vi "Operator error message space bar or print label.vi"(8 "error in (no error)":errorcluster, 11 "Message":string) -> (0 "error out":errorcluster, 3 "F1 Key hit?":bool)   [LabVIEW 2013]
uses:
  <vilib>/event_ctls.llb/eventvkey.ctl
panel:
  # "Operator Message"
  # "Press SPACE BAR to continue with no error label, else F1 key to print error label"
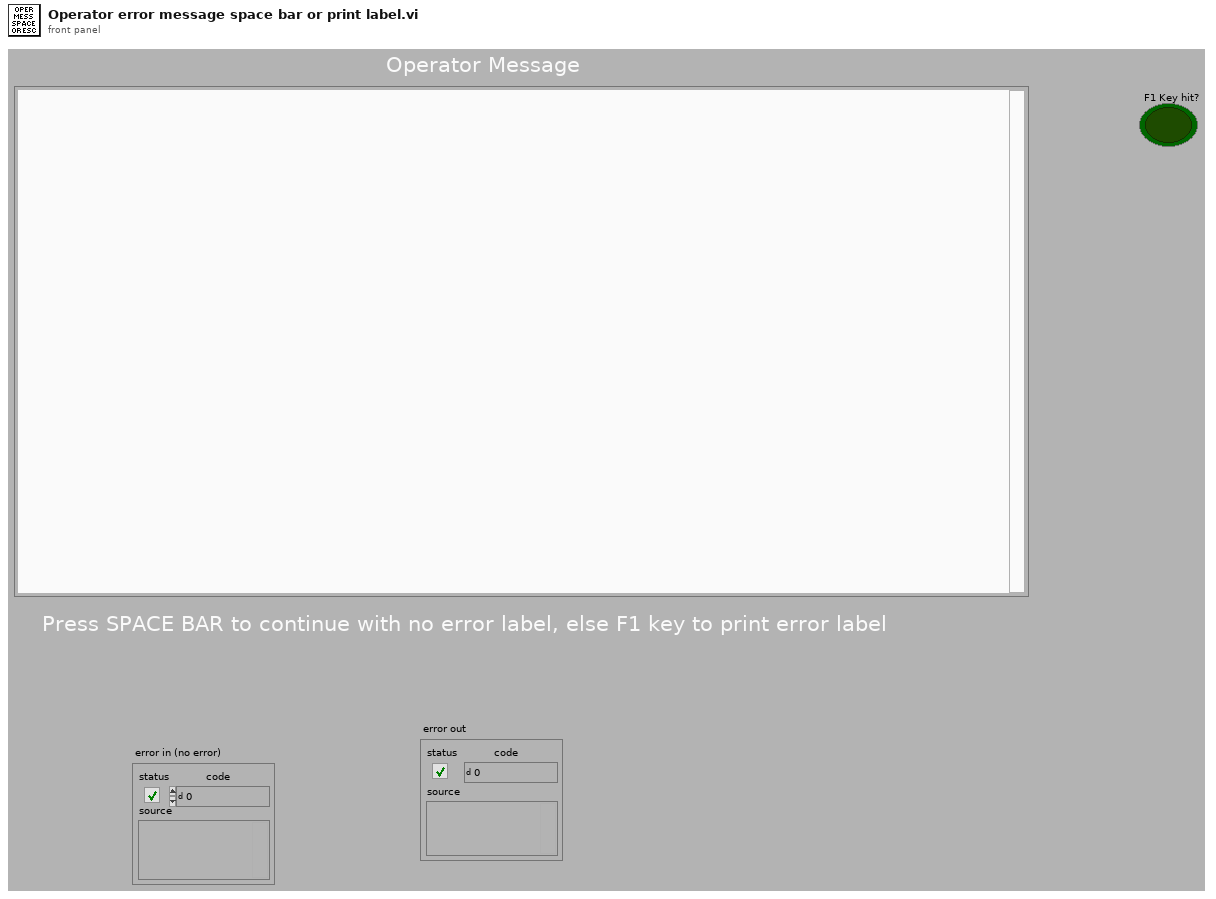
[diagram p1: front panel]
types:
  T1 = typedef "eventvkey.ctl" = enum16{"ASCII", "Enter", "Return", "Shift", "Ctrl", "Alt", "Cmd", "Opt", "Caps", "NumLock", "Clear", "Break", "Up", "Down", "Left", "Right", "Insert", "Delete", "Home", "End", "PageUp", "PageDown", "Escape", "Help", "Pause", "ScrollLock", "F1", "F2", "F3", "F4", "F5", "F6", "F7", "F8", "F9", "F10", "F11", "F12", "F13", "F14", "F15", "F16", "F17", "F18", "F19", "F20", "F21", "F22", "F23", "F24", "Play", "VolumeUp", "VolumeDown", "Mute", "Two Byte Char"}
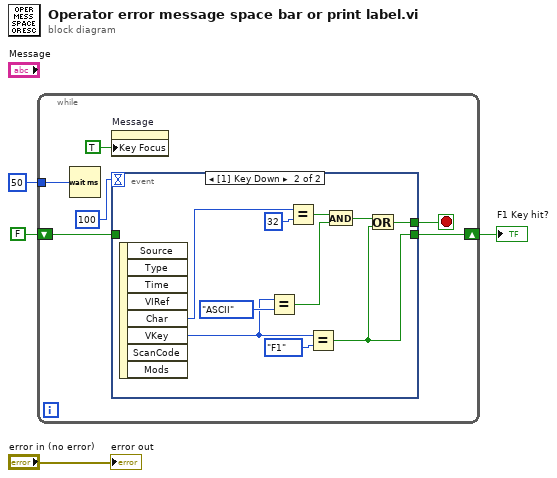
[diagram p0: block diagram]
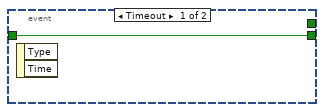
[diagram p2: hidden frame]
diagram:
  n1 = while {
    tunnel: u32 50 ("milliseconds to wait") -> [w10]
    shift-right: [w8] -> w2
    shift-left: FALSE -> [w7]
    stop <- w9 stop-if-true
    n2 = Wait (ms)(milliseconds to wait=w10) -> ()  [unwired: 1 out]
    n3 = property on="Message" class="Str"("Key Focus"=TRUE) -> ()  [unwired: 2 in, 2 out]
    n4 = event shown="[1] Key Down" {
      selector: _ -> [_ _]
      dyn-events: _ -> [_ _]
      timeout: 100 -> [_ _]
      tunnel: [_ w13] -> w9
      tunnel: [w11 w12] -> w8
      tunnel: w7 -> [w11 _]
      event Timeout {
        n5 = event-data() -> ()  [unwired: 1 in, 2 out]
      }
      event Key Down {
        n6 = event-data() -> ("Char"=w21:i16, "VKey"=w16:T1)  [unwired: 1 in, 6 out]
        n7 = Equal?(x=w16, y=eventvkey."ASCII" ("VKey")) -> (x = y?=w17:bool)
        n8 = Equal?(x=w21, y=i16 32) -> (x = y?=w18:bool)
        n9 = Equal?(x=w16, y=eventvkey."F1") -> (x = y?=w12:bool)
        n10 = And(x=w18, y=w17) -> (x .and. y?=w14:bool)
        n11 = Or(x=w14, y=w12) -> (x .or. y?=w13:bool)
      }
    }
  }
  "F1 Key hit?" <- w2
  "error out" <- "error in (no error)"
